vi "Get 2D Field (Cartesian).vi"(1 "Y-Axis Communications Config":T1={"GPIB address"=22, "GPIB bus"=0, "connection ID"=refnum, "IP"="192.168.2.200", "Active Comm Interface"=0, "Serial Port"="", "Programmer Type"=0} {"Programmer Type" items=["Model 430", "Model 420"]; "Active Comm Interface" items=["TCP/IP (Model 430 Only)", "RS232", "IEEE488"]}, 2 "Z-Axis Communications Config":T1={"GPIB address"=22, "GPIB bus"=0, "connection ID"=refnum, "IP"="192.168.2.200", "Active Comm Interface"=0, "Serial Port"="", "Programmer Type"=0} {"Programmer Type" items=["Model 430", "Model 420"]; "Active Comm Interface" items=["TCP/IP (Model 430 Only)", "RS232", "IEEE488"]}, 3 "error in":T2) -> (4 "All Instruments Responded?":bool, 6 "Y-Axis Field (kG)":dbl format="%.3f", 7 "Z-Axis Field (kG)":dbl format="%.3f", 8 "error out":T2)   [LabVIEW 2016]
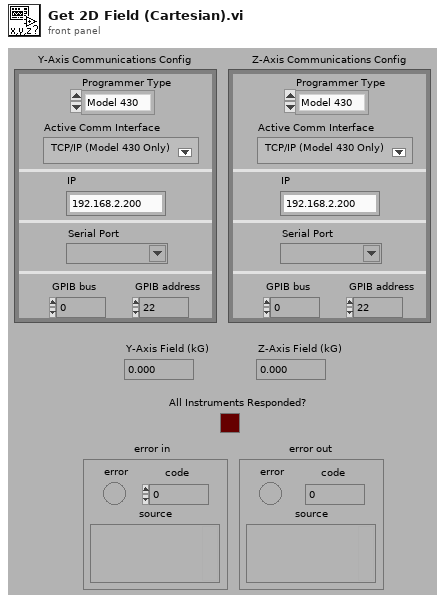
[diagram p1: front panel]
types:
  T1 = cluster{"GPIB address":i16, "GPIB bus":i16, "connection ID":refnum<k5>, "IP":string, "Active Comm Interface":u16, "Serial Port":refnum<visa-resource-name>, "Programmer Type":u16}
  T2 = cluster{"error":bool, "code":i32, "source":string}
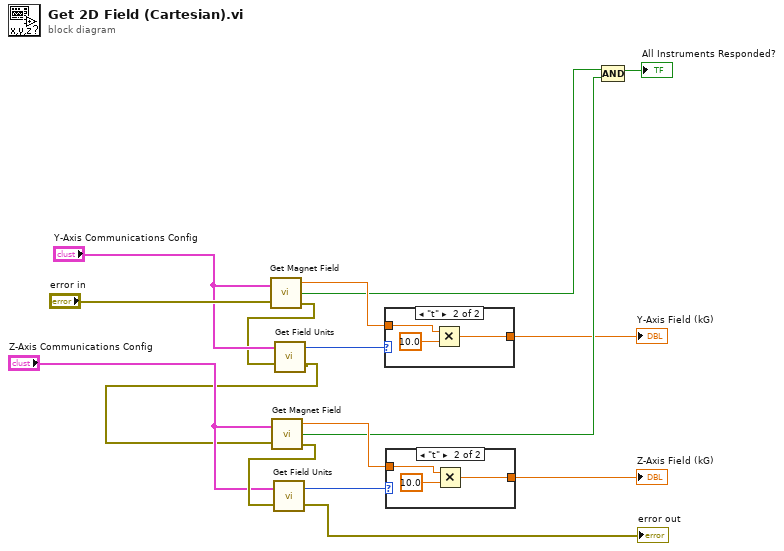
[diagram p0: block diagram]
diagram:
  n1 = call "Get Magnet Field.vi"("Communications Config"="Y-Axis Communications Config", "error in"="error in") -> ("Magnet Field (kG)"=w15:dbl, "Instrument Responded?"=w11:bool, "error out"=w3:T2)
  n2 = call "Get Field Units.vi"("error in"=w3, "Communications Config"="Y-Axis Communications Config") -> ("error out"=w2:T2, "Field Units"=w1:enum16{"kg", "t"})
  n3 = call "Get Magnet Field.vi"("Communications Config"="Z-Axis Communications Config", "error in"=w2) -> ("Magnet Field (kG)"=w12:dbl, "Instrument Responded?"=w10:bool, "error out"=w14:T2)
  n4 = call "Get Field Units.vi"("error in"=w14, "Communications Config"="Z-Axis Communications Config") -> ("error out"=→"error out":T2, "Field Units"=w13:enum16{"kg", "t"})
  n5 = case shown="\"t\"" w1 {
    tunnel: w15 -> [w17 w19]
    tunnel: [w17 w18] -> w7
    frame "kg", Default {
    }
    frame "t" {
      n6 = Multiply(x=w19, y=10.0) -> (x*y=w18:dbl)
    }
  }
  "Y-Axis Field (kG)" <- w7
  n7 = case shown="\"t\"" w13 {
    tunnel: w12 -> [w21 w23]
    tunnel: [w21 w22] -> w8
    frame "kg", Default {
    }
    frame "t" {
      n8 = Multiply(x=w23, y=10.0) -> (x*y=w22:dbl)
    }
  }
  "Z-Axis Field (kG)" <- w8
  n9 = Compound Arithmetic op=AND(w11, w10) -> (→"All Instruments Responded?":bool)
